vi "GPS仪器串口通讯.vi"(2 "输入指令":string, 3 "baud rate (9600)":u32=9600, 4 "VISA resource name":refnum<visa-resource-name>="COM3") -> (0 "read buffer":string, 1 "子字符串;substring":string)   [LabVIEW 2016]
uses:
  <vilib>/Instr/_visa.llb/VISA Configure Serial Port (Instr).vi
panel:
  out "输入的字符串":string
  out "返回数 2":u32
  out "返回数":u32
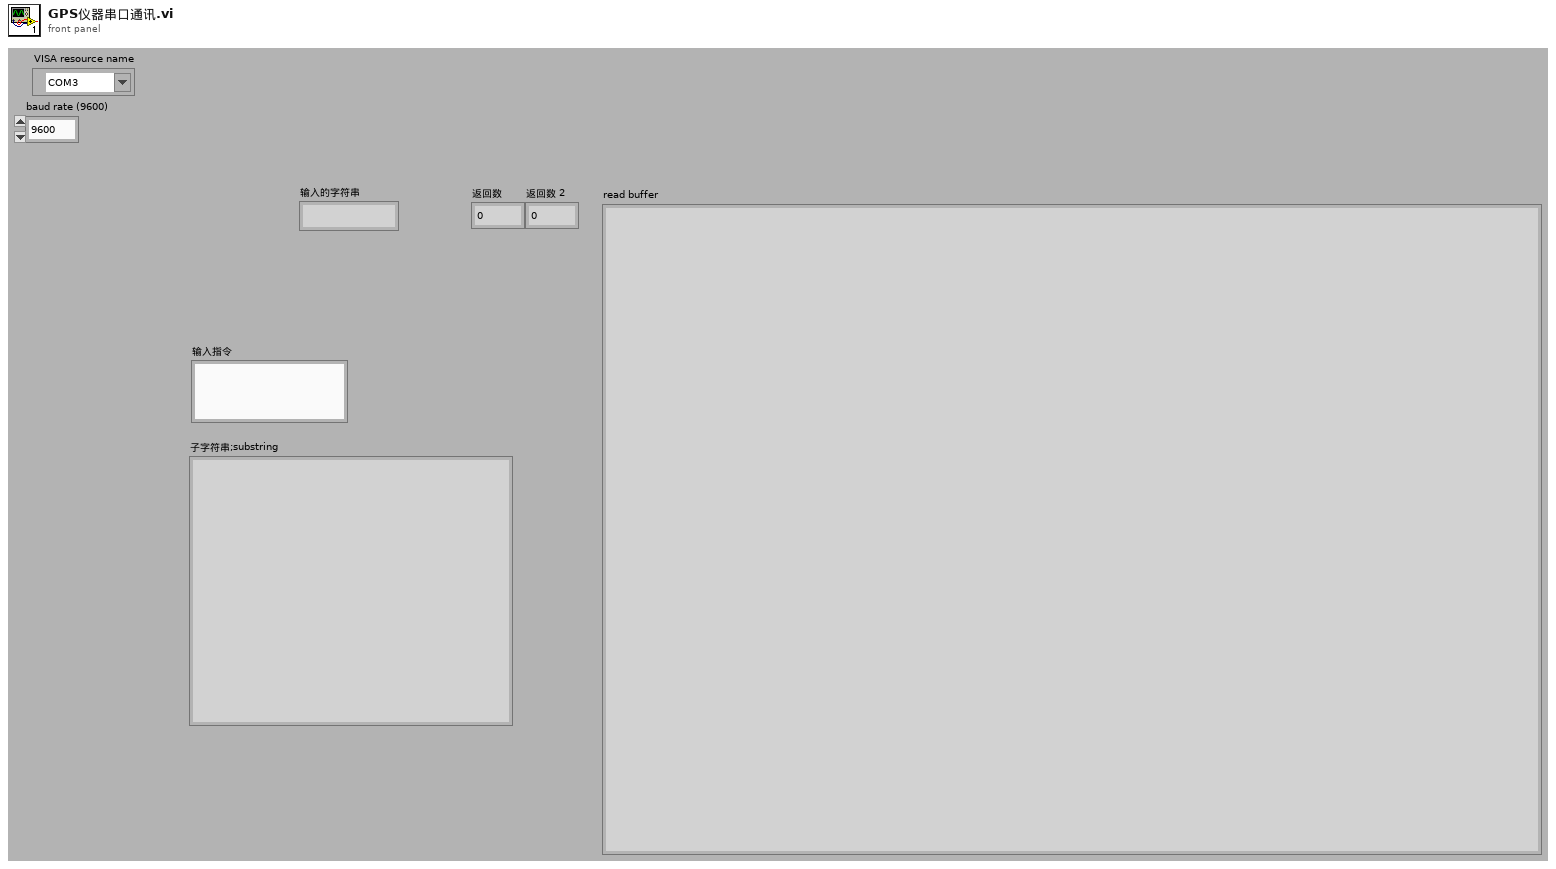
[diagram p1: front panel]
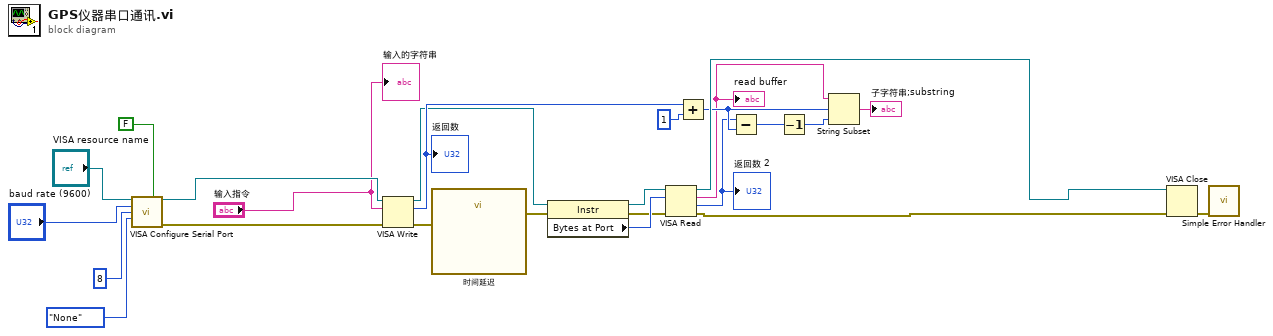
[diagram p0: block diagram]
diagram:
  n1 = call-poly "VISA Configure Serial Port"("VISA resource name"="VISA resource name", "Enable Termination\nChar (T)"=FALSE ("Enable Termination\nChar (T)"), "baud rate (9600)"="baud rate (9600)", "data bits (8)"=u16 8, "parity (0:none)"=enum16{"None", "Odd", "Even", "Mark", "Space"}."None") -> ("VISA resource name out"=w22:refnum<visa-resource-name>, "error out"=w21:errorcluster)  [unwired: 9 in]
  n2 = VISA Write(VISA resource name=w22, write buffer="输入指令", error in (no error)=w21) -> (VISA resource name out=w3:refnum<visa-resource-name>, return count=w8:u32, error out=w16:errorcluster)
  "返回数" <- w8
  n3 = call "时间延迟"("error in (no error)"=w16) -> ("error out"=w15:errorcluster)  [unwired: 10 in]
  n4 = property class="Instr"(reference=w3, error in=w15) -> (reference out=w12:refnum<visa-resource-name>, error out=w13:errorcluster, "Bytes at Port"=w14:u32)
  n5 = VISA Read(VISA resource name=w12, byte count=w14, error in (no error)=w13) -> (VISA resource name out=w19:refnum<visa-resource-name>, read buffer=w7:string, return count=w6:u32, error out=w20:errorcluster)
  "read buffer" <- w7
  "返回数 2" <- w6
  n6 = Add(x=w8, y=1 ("偏移量(0)")) -> (x+y=w10:u32)
  n7 = Subtract(x=w6, y=w10) -> (x-y=w4:u32)
  n8 = Decrement(x=w4) -> (x-1=w5:u32)
  n9 = String Subset(string=w7, offset (0)=w10, length (rest)=w5) -> (substring=→"子字符串;substring":string)
  n10 = VISA Close(VISA resource name=w19, error in (no error)=w20) -> (error out=w18:errorcluster)
  n11 = call <vilib>:"Simple Error Handler.vi"("error in (no error)"=w18) -> ()  [unwired: 4 in, 5 out]
  "输入的字符串" <- "输入指令"
